vi "PasswordSetting.vi"() -> ()   [LabVIEW 2024]
panel:
  out "String 2":string
  in  "Search Button":bool
  out "String":string
  out "Slide":u8(slide) scale=0.0..100.0
  in  "Password":T1
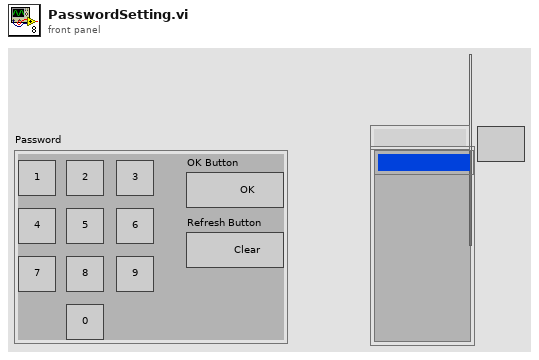
[diagram p1: front panel]
types:
  T1 = cluster{"Blank Button":bool, "Blank Button 2":bool, "Blank Button 3":bool, "Blank Button 4":bool, "Blank Button 5":bool, "Blank Button 6":bool, "Blank Button 7":bool, "Blank Button 8":bool, "Blank Button 9":bool, "Blank Button 10":bool, "OK Button":bool, "Refresh Button":bool}
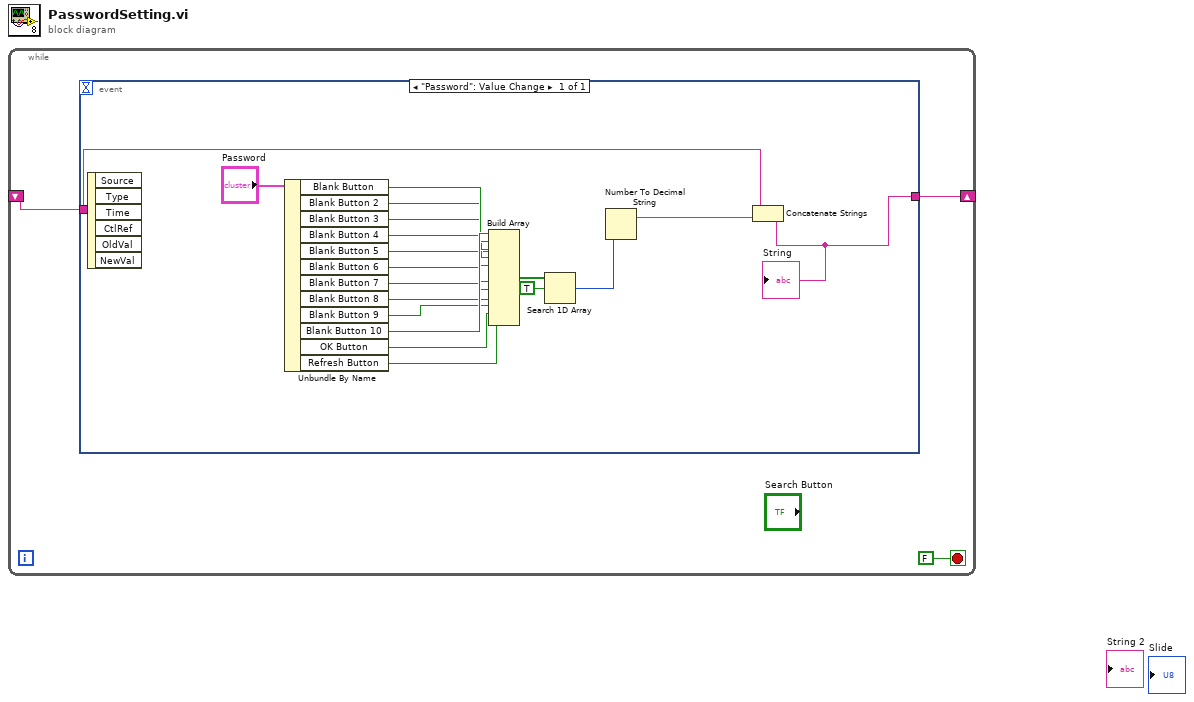
[diagram p0: block diagram]
diagram:
  n1 = while {
    shift-right: [w2] -> _
    shift-left: _ -> [w1]
    stop <- FALSE stop-if-true
    n2 = event shown="[0] \"Password\": Value Change" {
      selector: _ -> [_]
      dyn-events: _ -> [_]
      timeout: _ -> [_]
      tunnel: [w6] -> w2
      tunnel: w1 -> [w4]
      event "Password": Value Change {
        n3 = event-data() -> ()  [unwired: 1 in, 6 out]
        n4 = Unbundle By Name "Unbundle By Name"("Password") -> ("Blank Button"=w20:bool, "Blank Button 2"=w19:bool, "Blank Button 3"=w18:bool, "Blank Button 4"=w17:bool, "Blank Button 5"=w16:bool, "Blank Button 6"=w15:bool, "Blank Button 7"=w14:bool, "Blank Button 8"=w13:bool, "Blank Button 9"=w12:bool, "Blank Button 10"=w21:bool, "OK Button"=w11:bool, "Refresh Button"=w10:bool)
        n5 = Build Array "Build Array"(w21, w20, w19, w18, w17, w16, w15, w14, w13, w12, w11, w10) -> (w9:bool[])
        n6 = Search 1D Array(1D array=w9, element=TRUE) -> (index of element=w7:i32)  [unwired: 1 in]
        n7 = Number To Decimal String(number=w7) -> (decimal integer string=w5:string)  [unwired: 1 in]
        n8 = Concatenate Strings(w4, w5) -> (w6:string)
        "String" <- w6
      }
    }
  }
